vi "FGV Ergebnis.vi"(6 "Enum":T3, 8 "Bestanden?":bool, 9 "Graph":waveform(dbl)[][](array[waveform]), 10 "Interference Daten":T2 {"Target Conc. 3" format="%#_5g"; "Target Conc 2" format="%#_5g"; "Target conc." format="%#_5g"; "Flow-weighted mean" format="%#_5g"}, 11 "Wasserkonz":sgl) -> (0 "Protokoll":T1[](array[typedef]), 1 "Interference Daten":T2 {"Target Conc. 3" format="%#_5g"; "Target Conc 2" format="%#_5g"; "Target conc." format="%#_5g"; "Flow-weighted mean" format="%#_5g"}, 2 "Graph":waveform(dbl)[][](array[waveform]), 3 "Wasserkonz":sgl, 4 "Zeitstempel":string, 5 "Bestanden?":bool)   [LabVIEW 2020, in "EPA 1065.lvlib" / "HovaCAL Interference verificaton.lvlib"]
uses:
  HovaCAL Interference verificaton.lvlib
  Seiten/FT-IR/FT-IR.lvlib
  Seiten/FT-IR/FGV FT-IR Gasliste Aktionen.ctl
  Seiten/Gaszuordnung AO/Gaszuordnung AO.lvlib
  Seiten/Gaszuordnung AO/FGV Gaszuordnung Grenzen&Einheit Aktion.ctl
  Visualisierungs Elemente/String - Ausgabefeld.ctl
  Sprachverwaltung/Sprachverwaltung.lvlib
  Sprachverwaltung/FGV Aktion Tabelle zerlegen.ctl
  Aktion FGV Test.ctl
  Interference Daten.ctl
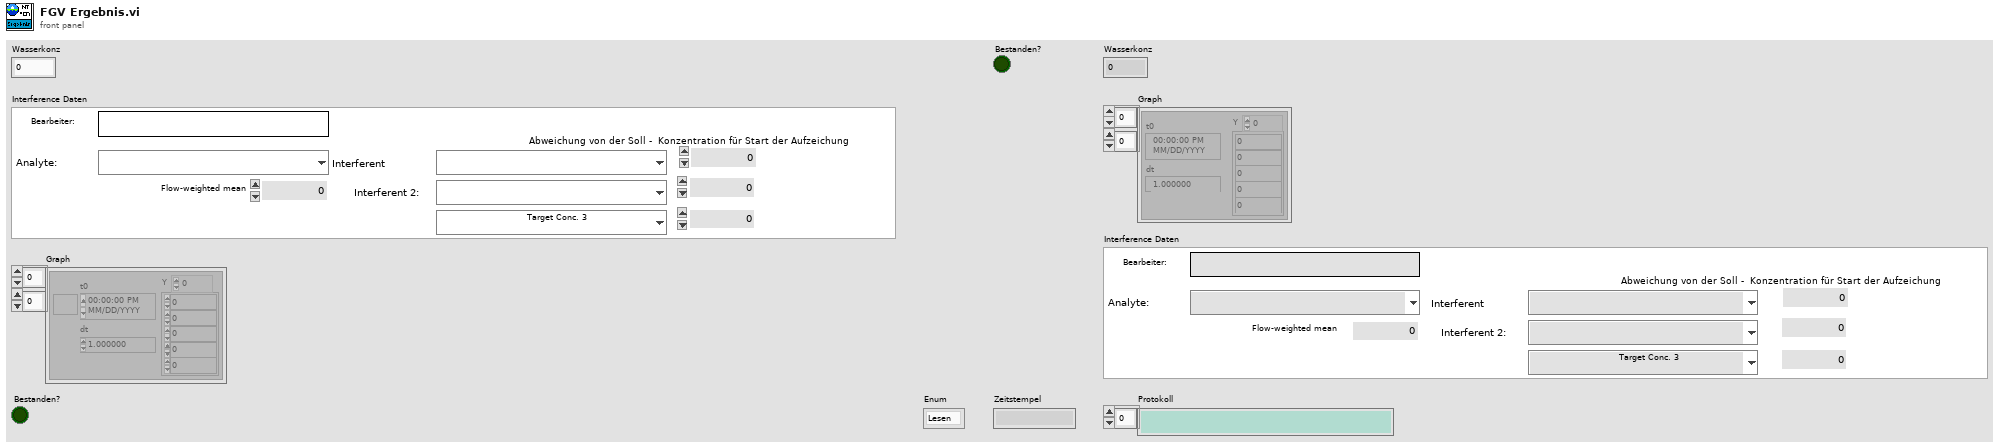
[diagram p1: front panel]
types:
  T1 = typedef "String - Ausgabefeld.ctl" = string
  T2 = typedef "EPA 1065.lvlib/HovaCAL Interference verificaton.lvlib/Interference Daten.ctl" = cluster{"Bearbeiter:":string, "Analyte:":u16, "Flow-weighted mean":sgl, "Target conc.":sgl, "Interferent":u16, "Interferent 2:":u16, "Interferent 3:":u16, "Target Conc 2":sgl, "Target Conc. 3":sgl}
  T3 = typedef "EPA 1065.lvlib/HovaCAL Interference verificaton.lvlib/Aktion FGV Test.ctl" = enum16{"Lesen", "ini", "Wasserkonzentration", "Wet", "Dry", "Ergebnis", "Graph", "Interference Daten", "Speichern"}
  T4 = typedef "Sprachverwaltung.lvlib/FGV Aktion Tabelle zerlegen.ctl" = enum16{"laden", "vereinzeln", "speichern"}
  T5 = typedef "Gaszuordnung AO.lvlib/FGV Gaszuordnung Grenzen&Einheit Aktion.ctl" = enum16{"Lesen", "Schreiben Min", "Schreiben Max", "Laden", "Speichern"}
  T6 = typedef "FT-IR.lvlib/FGV FT-IR Gasliste Aktionen.ctl" = enum16{"lesen", "Gasliste FT-IR", "Gasliste ausgelesen", "laden", "speichern", "löschen"}
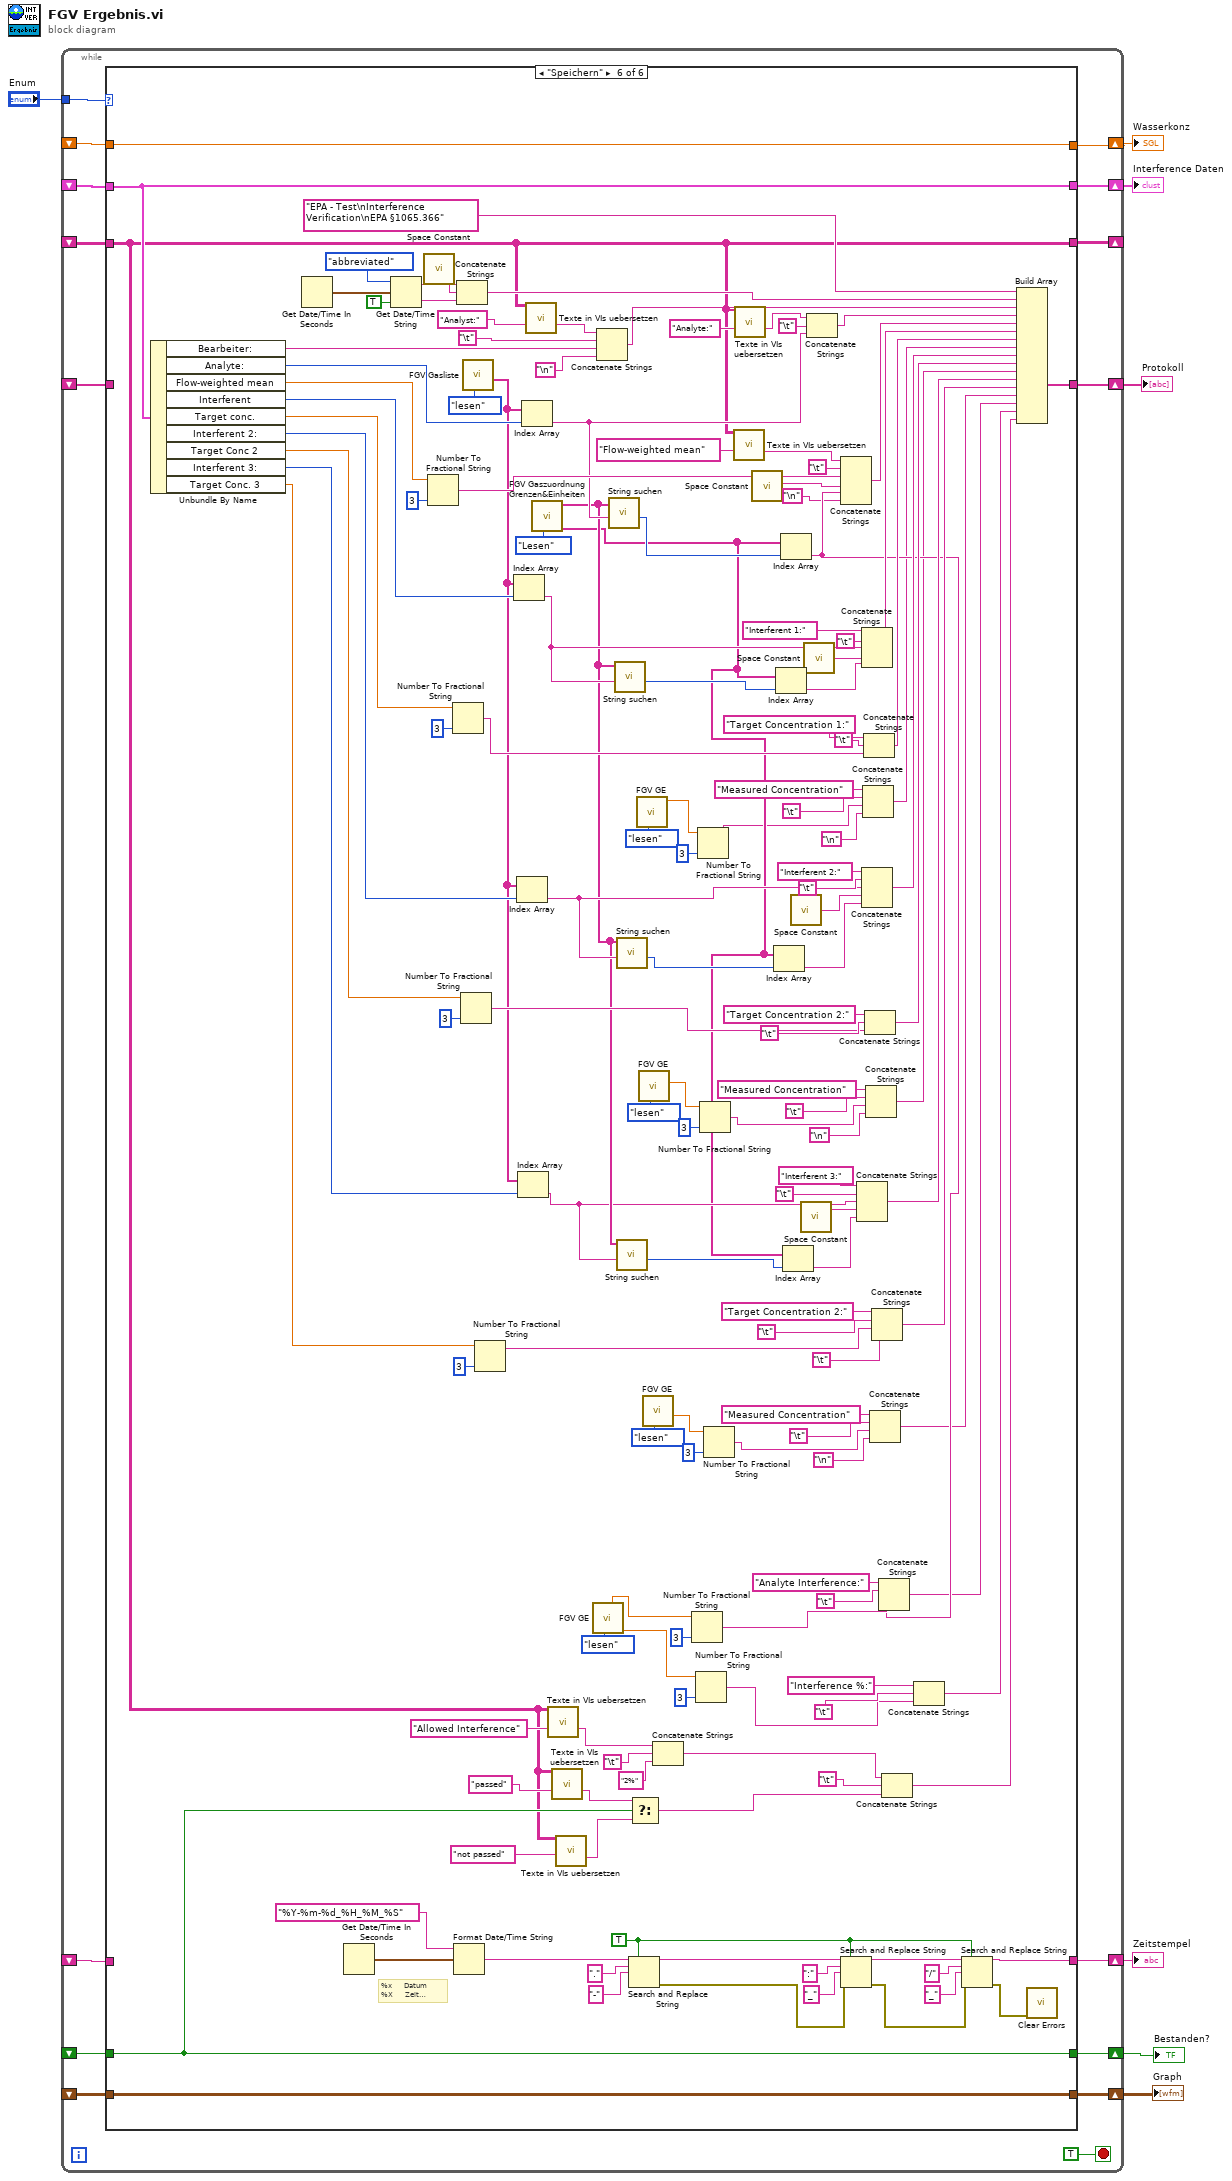
[diagram p0: block diagram]
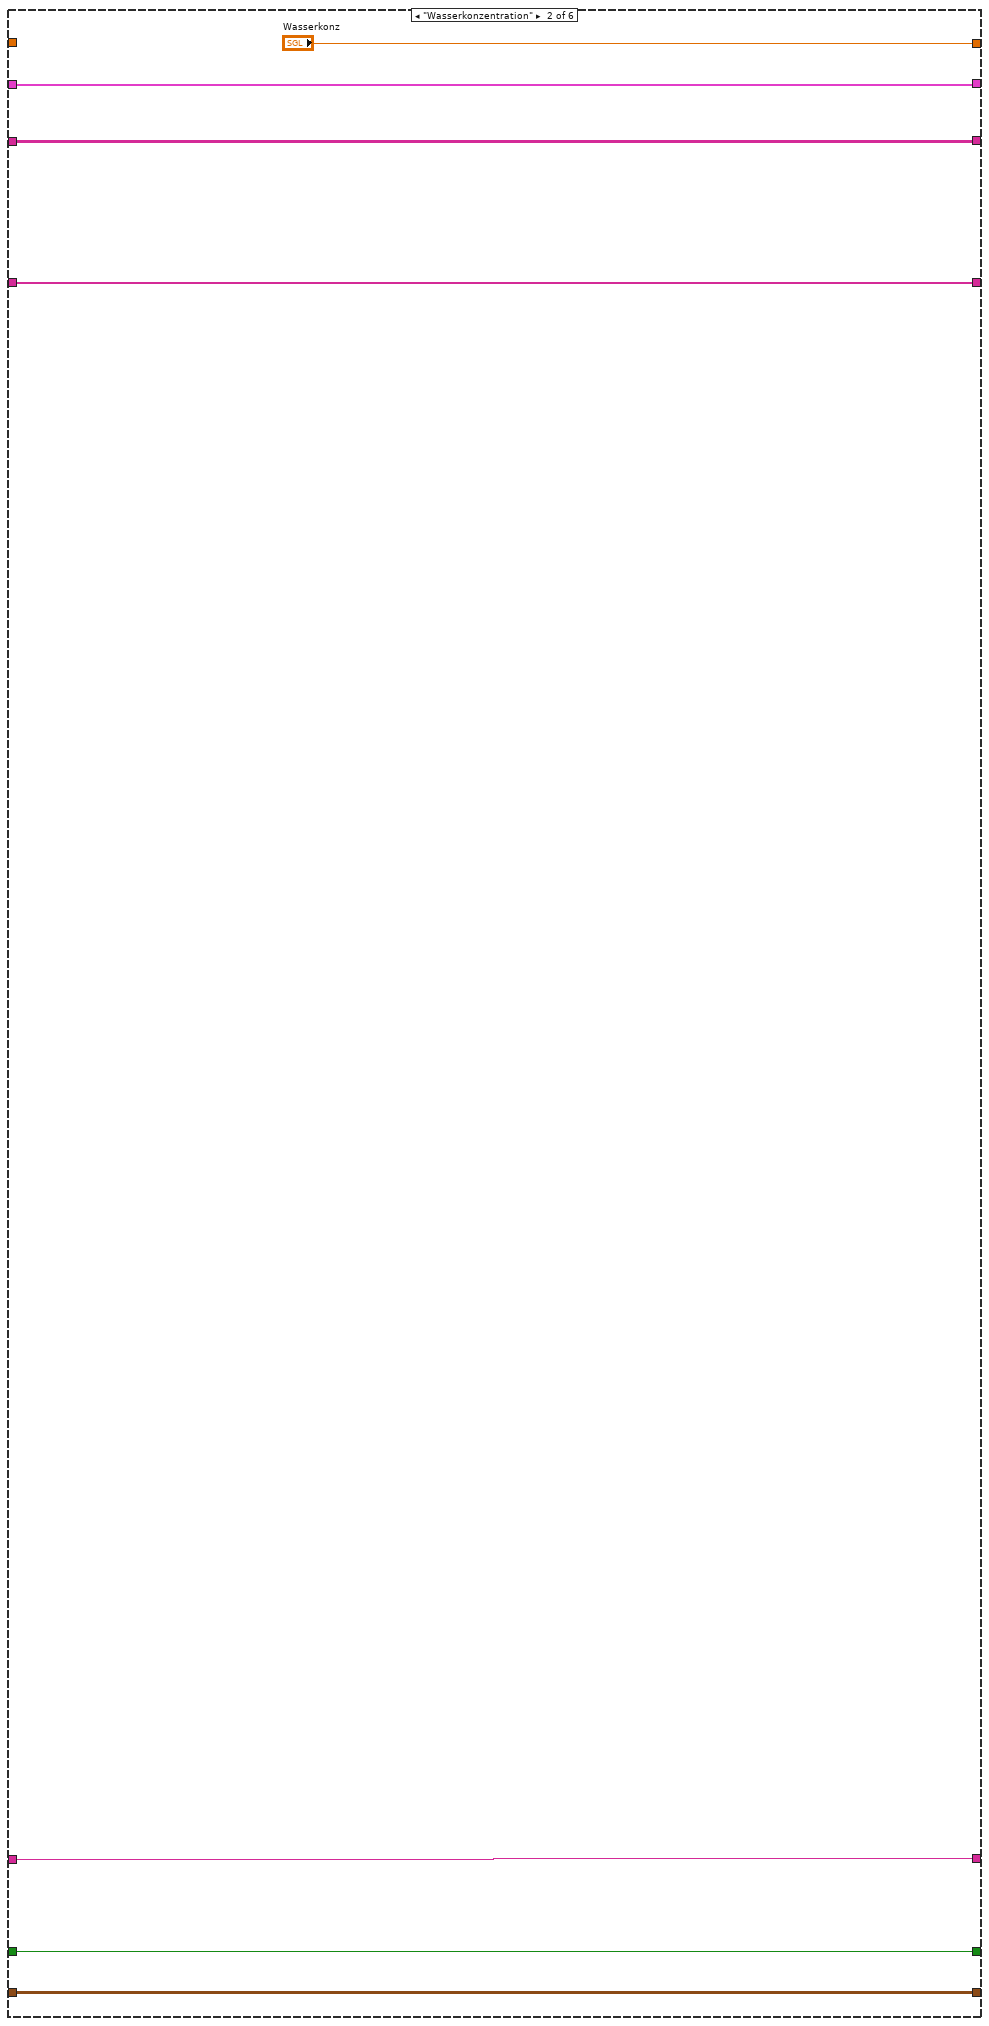
[diagram p3: hidden frame]
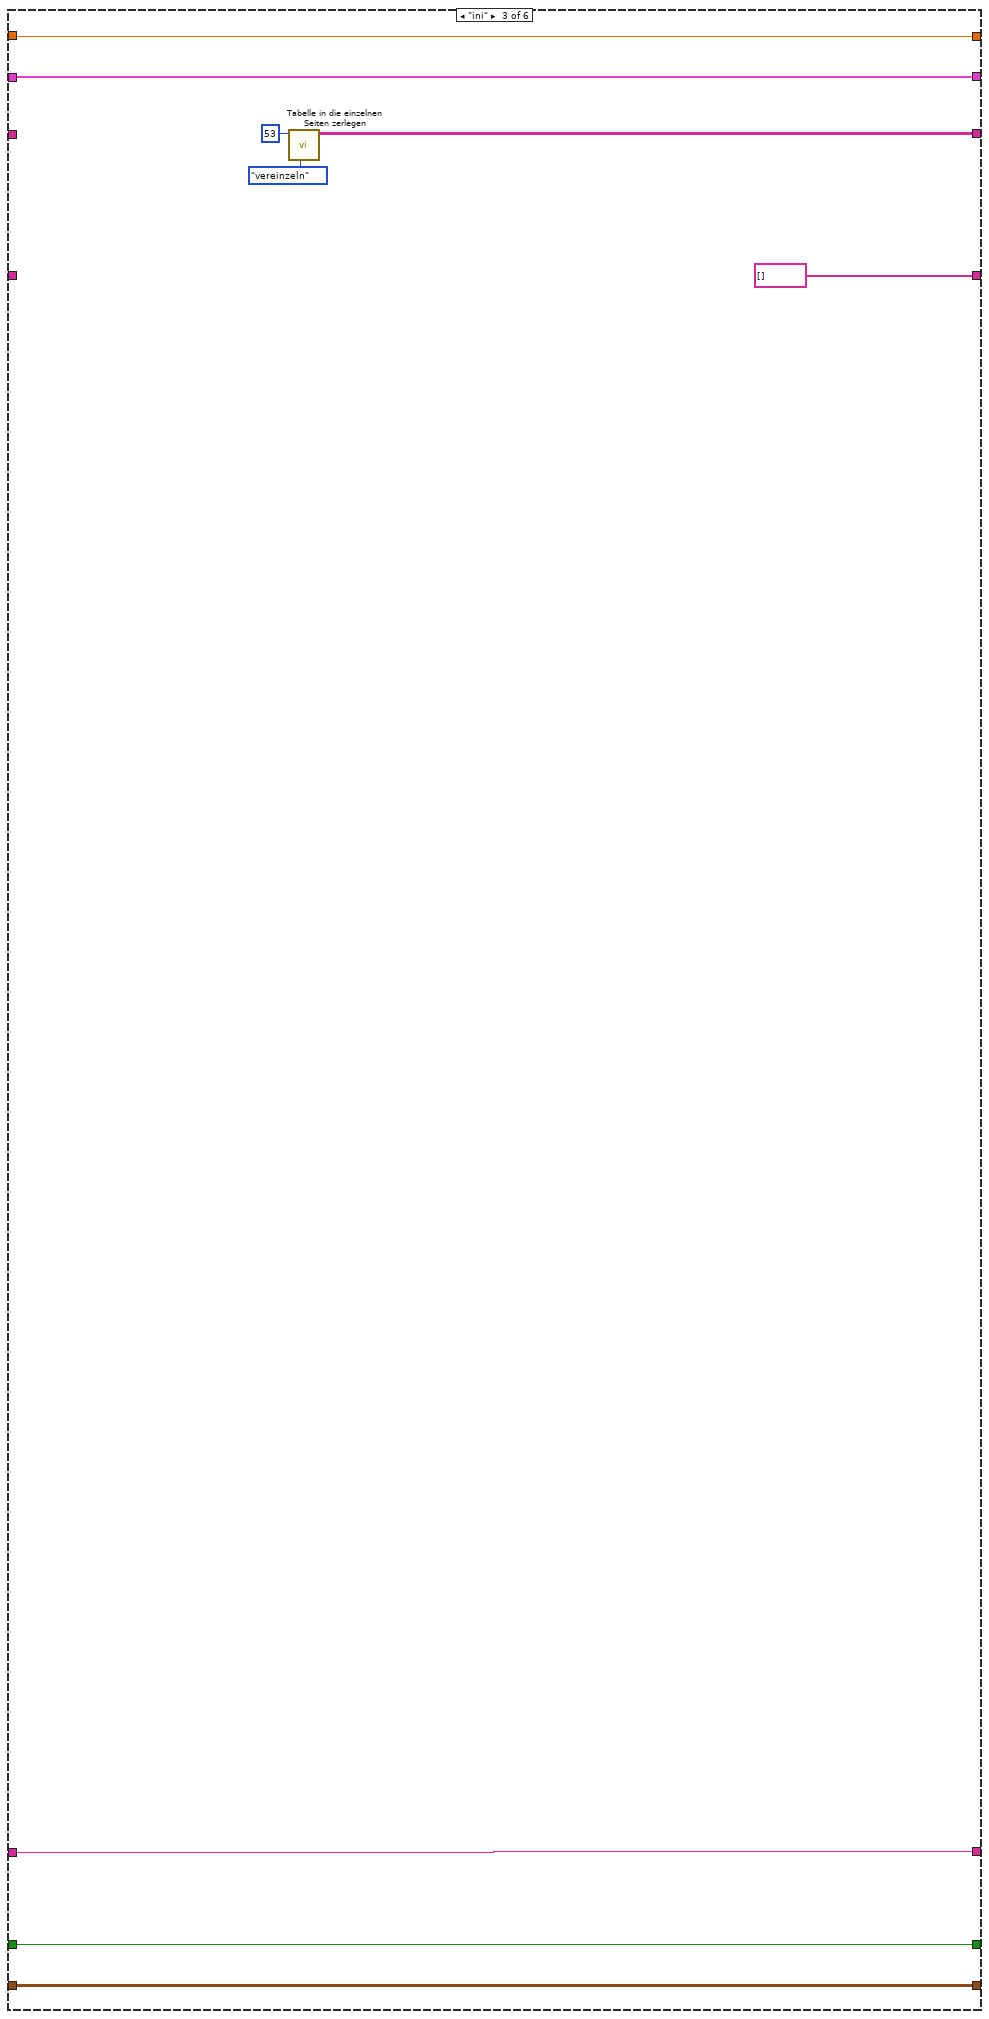
[diagram p4: hidden frame]
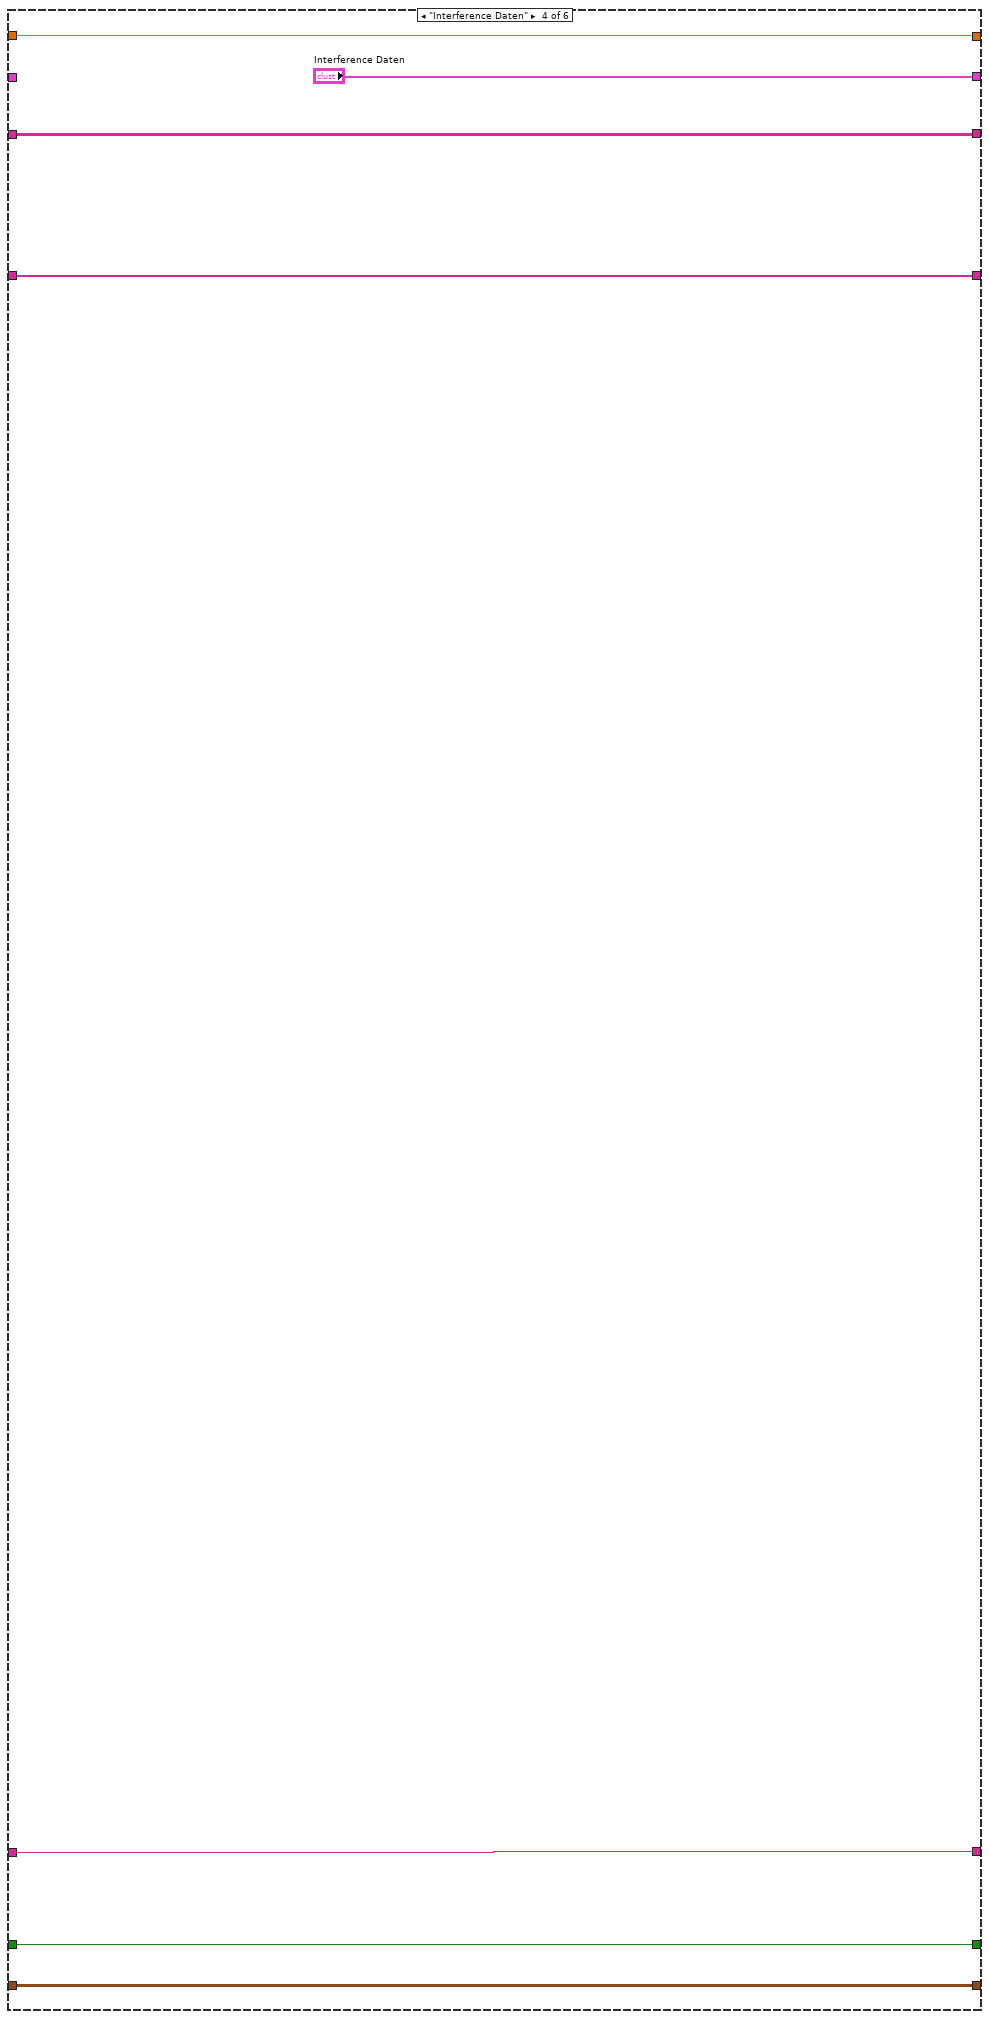
[diagram p5: hidden frame]
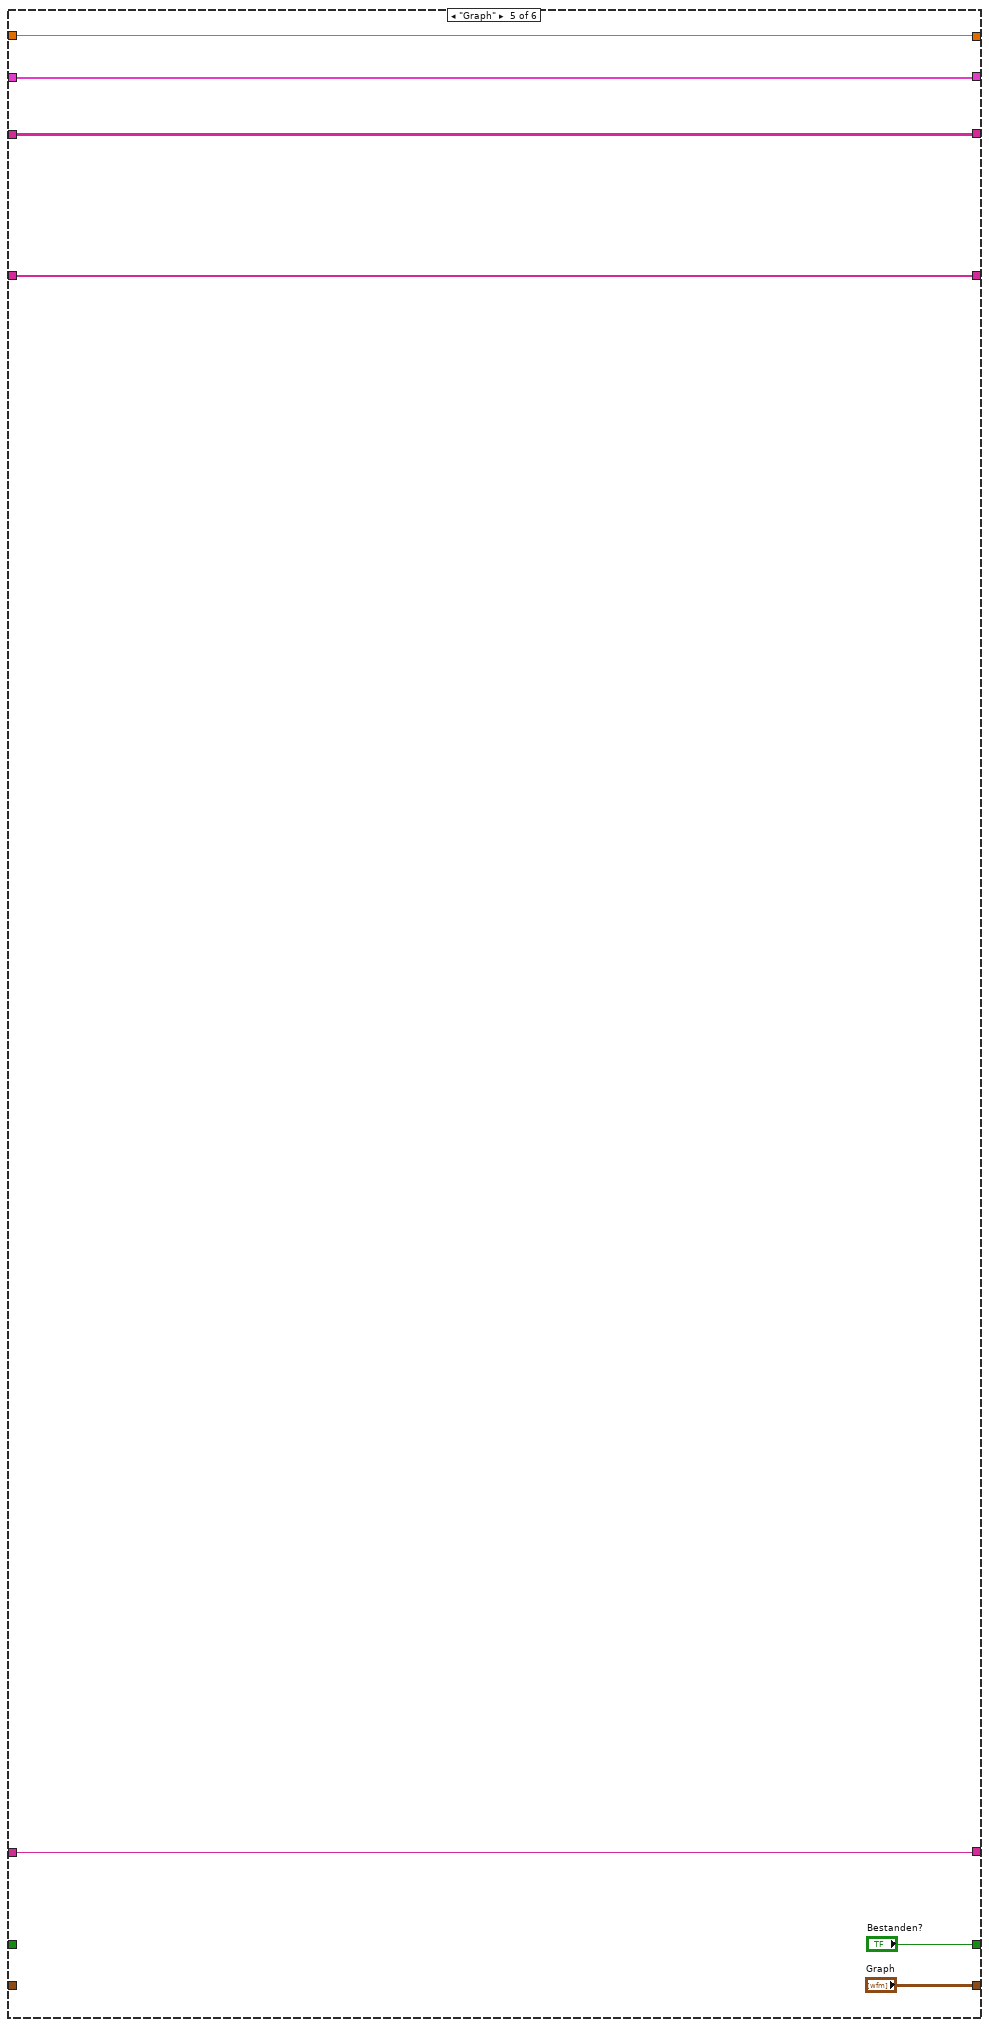
[diagram p6: hidden frame]
diagram:
  n1 = while {
    tunnel: "Enum" -> [w22]
    shift-right: [w21] -> w6
    shift-left: _ -> [w20]
    shift-right: [w14] -> w5
    shift-left: _ -> [w19]
    shift-right: [w18] -> w1
    shift-left: _ -> [w17]
    shift-right: [w16] -> w4
    shift-left: _ -> [w15]
    shift-right: [w13] -> w3
    shift-left: _ -> [w12]
    shift-right: [w11] -> w2
    shift-left: _ -> [w10]
    shift-right: [w8] -> _
    shift-left: _ -> [w9]
    stop <- TRUE stop-if-true
    n2 = case shown="\"Speichern\"" w22 {
      tunnel: [w30 "Wasserkonz" w45 w53 w59 w189] -> w21
      tunnel: w20 -> [w30 _ w45 w53 w59 w189]
      tunnel: [w29 w36 w41 "Interference Daten" w58 w204] -> w14
      tunnel: w19 -> [w29 w36 w41 _ w58 w204]
      tunnel: [w28 w35 T1[] [] w51 w57 w188] -> w18
      tunnel: w17 -> [w28 w35 _ w51 w57 _]
      tunnel: [w27 w34 w44 w50 w60 w170] -> w16
      tunnel: w15 -> [w27 w34 w44 w50 w60 _]
      tunnel: [w26 w33 w43 w49 "Graph" w168] -> w13
      tunnel: w12 -> [w26 w33 w43 w49 _ w168]
      tunnel: [w25 w32 w42 w48 "Bestanden?" w95] -> w11
      tunnel: w10 -> [w25 w32 w42 w48 _ w95]
      tunnel: w9 -> [w24 w31 _ w47 w54 w94]
      tunnel: [w24 w31 w38 w47 w54 w94] -> w8
      frame "Lesen", Default {
      }
      frame "Wasserkonzentration" {
      }
      frame "ini" {
        n3 = call "Tabelle in die einzelnen Seiten zerlegen.vi"("Aktion"=FGV_Aktion_Tabelle_zerlegen."vereinzeln", "Index (Seite)"=53) -> ("Sprachliste"=w38:string[][])  [unwired: 7 in, 2 out]
      }
      frame "Interference Daten" {
      }
      frame "Graph" {
      }
      frame "Speichern" {
        w171 = TRUE ("Alle ersetzen? (F)")
        # "%x      Datum\n%X      Zeit (h:m:s)"
        n4 = Unbundle By Name(w204) -> ("Bearbeiter:"=w202:string, "Analyte:"=w200:u16, "Flow-weighted mean"=w196:sgl, "Interferent"=w161:u16, "Target conc."=w153:sgl, "Interferent 2:"=w147:u16, "Target Conc 2"=w140:sgl, "Interferent 3:"=w133:u16, "Target Conc. 3"=w123:sgl)
        n5 = Get Date/Time In Seconds() -> (seconds since 1Jan1904=w205:timestamp)
        n6 = Get Date/Time In Seconds() -> (seconds since 1Jan1904=w185:timestamp)
        n7 = Get Date/Time String(date format (0)=enum16{"short", "long", "abbreviated"}."abbreviated" ("Datumsformat (0)"), seconds (now)=w205, want seconds? (F)=TRUE ("Angabe von Sekunden? (F)")) -> (date string=w208:string, time string=w210:string)
        n8 = call <vilib>:"Space Constant.vi"() -> ("String"=w209:string)
        n9 = Number To Fractional String(number=w196, precision (6)=i16 3 ("Genauigkeit (6)")) -> (F-format string=w194:string)  [unwired: 2 in]
        n10 = Number To Fractional String(number=w153, precision (6)=i16 3 ("Genauigkeit (6)")) -> (F-format string=w152:string)  [unwired: 2 in]
        n11 = Format Date/Time String(time format string (%c)="%Y-%m-%d_%H_%M_%S" ("Zeitformatierungs-String (%c)"), seconds (now)=w185) -> (date/time string=w184:string)  [unwired: 1 in]
        n12 = Concatenate Strings(w208, w209, w210) -> (w198:string)
        n13 = Number To Fractional String(number=w140, precision (6)=i16 3 ("Genauigkeit (6)")) -> (F-format string=w139:string)  [unwired: 2 in]
        n14 = call "FGV Gasliste.vi"("Aktionen"=FGV_FT-IR_Gasliste_Aktionen."lesen") -> ("Aktuelle Gasliste gesamt"=w64:T1[])  [unwired: 8 in, 2 out]
        n15 = Number To Fractional String(number=w123, precision (6)=i16 3 ("Genauigkeit (6)")) -> (F-format string=w122:string)  [unwired: 2 in]
        n16 = Index Array(array=w64, index=w161) -> (element=w134:T1)
        n17 = Index Array(array=w64, index=w147) -> (element=w146:T1)
        n18 = Index Array(array=w64, index=w133) -> (element=w131:T1)
        n19 = Index Array(array=w64, index=w200) -> (element=w187:T1)
        n20 = call "Texte in VIs uebersetzen.vi"("Sprachliste"=w94, "String zum Übersetzen"="Analyst:" ("String")) -> ("String zum Übersetzen"=w164:string)  [unwired: 9 in, 4 out]
        n21 = call "FGV Gaszuordnung Grenzen&Einheiten.vi"("Aktion"=FGV_Gaszuordnung_Grenzen&Einheit_Aktion."Lesen") -> ("Einheit neu"=w130:string[], "Namen neu"=w132:string[])  [unwired: 2 in, 7 out]
        n22 = call "Texte in VIs uebersetzen.vi"("Sprachliste"=w94, "String zum Übersetzen"="Allowed Interference" ("String")) -> ("String zum Übersetzen"=w116:string)  [unwired: 9 in, 4 out]
        n23 = call "Texte in VIs uebersetzen.vi"("Sprachliste"=w94, "String zum Übersetzen"="passed" ("String")) -> ("String zum Übersetzen"=w114:string)  [unwired: 9 in, 4 out]
        n24 = call "Texte in VIs uebersetzen.vi"("Sprachliste"=w94, "String zum Übersetzen"="not passed" ("String")) -> ("String zum Übersetzen"=w112:string)  [unwired: 9 in, 4 out]
        n25 = call "FGV GE.vi"("Enum"=enum16{"lesen", "schreiben"}."lesen") -> ("Ergebnis %"=w103:sgl, "Ergebnis"=w108:sgl)  [unwired: 6 in, 3 out]
        n26 = Concatenate Strings(w164, "\t", w202, "\n") -> (w197:string)
        n27 = call "String suchen.vi"("Gasname"=w187, "Such-Namen"=w132) -> ("Index"=w192:i32)  [unwired: 8 in, 1 out]
        n28 = call "String suchen.vi"("Gasname"=w134, "Such-Namen"=w132) -> ("Index"=w158:i32)  [unwired: 8 in, 1 out]
        n29 = call "String suchen.vi"("Gasname"=w146, "Such-Namen"=w132) -> ("Index"=w145:i32)  [unwired: 8 in, 1 out]
        n30 = call "String suchen.vi"("Gasname"=w131, "Such-Namen"=w132) -> ("Index"=w129:i32)  [unwired: 8 in, 1 out]
        n31 = Search and Replace String(replace all?=w171, input string=w184, search string="." ("Such-String"), replace string="-" ("String ersetzen(\"\")")) -> (result string=w181:string, error out=w175:errorcluster)  [unwired: 4 in, 2 out]
        n32 = Select(t=w114, s=w95, f=w112) -> (s? t:f=w98:string)
        n33 = call "FGV GE.vi"("Enum"=enum16{"lesen", "schreiben"}."lesen") -> ("Inter1"=w87:sgl)  [unwired: 6 in, 4 out]
        n34 = call "FGV GE.vi"("Enum"=enum16{"lesen", "schreiben"}."lesen") -> ("Inter 2"=w79:sgl)  [unwired: 6 in, 4 out]
        n35 = call "FGV GE.vi"("Enum"=enum16{"lesen", "schreiben"}."lesen") -> ("Inter 3"=w72:sgl)  [unwired: 6 in, 4 out]
        n36 = Concatenate Strings(w116, "\t", "2%" ("String")) -> (w99:string)
        n37 = Number To Fractional String(number=w108, precision (6)=i16 3 ("Genauigkeit (6)")) -> (F-format string=w107:string)  [unwired: 2 in]
        n38 = Number To Fractional String(number=w103, precision (6)=i16 3 ("Genauigkeit (6)")) -> (F-format string=w100:string)  [unwired: 2 in]
        n39 = Number To Fractional String(number=w87, precision (6)=i16 3 ("Genauigkeit (6)")) -> (F-format string=w86:string)  [unwired: 2 in]
        n40 = Number To Fractional String(number=w79, precision (6)=i16 3 ("Genauigkeit (6)")) -> (F-format string=w81:string)  [unwired: 2 in]
        n41 = Number To Fractional String(number=w72, precision (6)=i16 3 ("Genauigkeit (6)")) -> (F-format string=w76:string)  [unwired: 2 in]
        n42 = call "Texte in VIs uebersetzen.vi"("Sprachliste"=w94, "String zum Übersetzen"="Flow-weighted mean") -> ("String zum Übersetzen"=w162:string)  [unwired: 9 in, 4 out]
        n43 = call "Texte in VIs uebersetzen.vi"("Sprachliste"=w94, "String zum Übersetzen"=T1 "Analyte:" ("Element")) -> ("String zum Übersetzen"=w166:string)  [unwired: 9 in, 4 out]
        n44 = call <vilib>:"Space Constant.vi"() -> ("String"=w69:string)
        n45 = Index Array(array=w130, index=w145) -> (element=w144:string)
        n46 = Index Array(array=w130, index=w158) -> (element=w157:string)
        n47 = Index Array(array=w130, index=w192) -> (element=w106:string)
        n48 = Index Array(array=w130, index=w129) -> (element=w128:string)
        n49 = call <vilib>:"Space Constant.vi"() -> ("String"=w67:string)
        n50 = call <vilib>:"Space Constant.vi"() -> ("String"=w66:string)
        n51 = call <vilib>:"Space Constant.vi"() -> ("String"=w68:string)
        n52 = Concatenate Strings(w166, "\t", w187) -> (w186:string)
        n53 = Concatenate Strings(w162, "\t", w194, w69, w106, "\n") -> (w191:string)
        n54 = Search and Replace String(replace all?=w171, input string=w181, search string=":" ("Such-String"), replace string="_" ("String ersetzen(\"\")"), error in=w175) -> (result string=w176:string, error out=w174:errorcluster)  [unwired: 3 in, 2 out]
        n55 = Concatenate Strings("Interferent 3:" ("String"), "\t", w131, w66, w128) -> (w127:string)
        n56 = Concatenate Strings("Interferent 1:" ("String"), "\t", w134, w68, w157) -> (w151:string)
        n57 = Concatenate Strings("Interferent 2:" ("String"), "\t", w146, w67, w144) -> (w138:string)
        n58 = Concatenate Strings("Measured Concentration" ("String"), "\t", w86, "\n") -> (w85:string)
        n59 = Concatenate Strings("Target Concentration 1:" ("String"), "\t", w152) -> (w150:string)
        n60 = Concatenate Strings("Target Concentration 2:" ("String"), "\t", w139) -> (w137:string)
        n61 = Concatenate Strings("Measured Concentration" ("String"), "\t", w81, "\n") -> (w71:string)
        n62 = Concatenate Strings("Measured Concentration" ("String"), "\t", w76, "\n") -> (w70:string)
        n63 = Concatenate Strings("Target Concentration 2:" ("String"), "\t", w122, "\t") -> (w121:string)
        n64 = Concatenate Strings("Analyte Interference:" ("String"), "\t", w107, w106) -> (w105:string)
        n65 = Concatenate Strings(w99, "\t", w98) -> (w65:string)
        n66 = Concatenate Strings("Interference %:" ("String"), "\t", w100) -> (w96:string)
        n67 = Search and Replace String(replace all?=w171, input string=w176, search string="/" ("Such-String"), replace string="_" ("String ersetzen(\"\")"), error in=w174) -> (result string=w170:string, error out=w173:errorcluster)  [unwired: 3 in, 2 out]
        n68 = Build Array("EPA - Test\nInterference Verification\nEPA §1065.366", w198, w197, w186, w191, w151, w150, w85, w138, w137, w71, w127, w121, w70, w105, w96, w65) -> (w188:string[])
        n69 = call <vilib>:"Clear Errors.vi"("error in (no error)"=w173) -> ()  [unwired: 5 in, 2 out]
      }
    }
  }
  "Wasserkonz" <- w6
  "Interference Daten" <- w5
  "Protokoll" <- w1
  "Zeitstempel" <- w4
  "Graph" <- w3
  "Bestanden?" <- w2
